vi "get_com_port.vi"(8 "error in (no error)":errorcluster, 11 "LightSourceAN191011Chameleon in":refnum<class "LightSourceAN191011Chameleon.lvclass">) -> (0 "error out":errorcluster, 2 "comm port":refnum<visa-resource-name>, 3 "LightSourceAN191011Chameleon out":refnum<class "LightSourceAN191011Chameleon.lvclass">)   [LabVIEW 2010, in "LightSourceAN191011Chameleon.lvclass"]
uses:
  LightSourceAN191011Chameleon.lvclass
  LightSourceAN191011Chameleon.lvclass/LightSourceAN191011Chameleon.ctl
  <vilib>/Instr/_visa.llb/VISA Configure Serial Port (Instr).vi
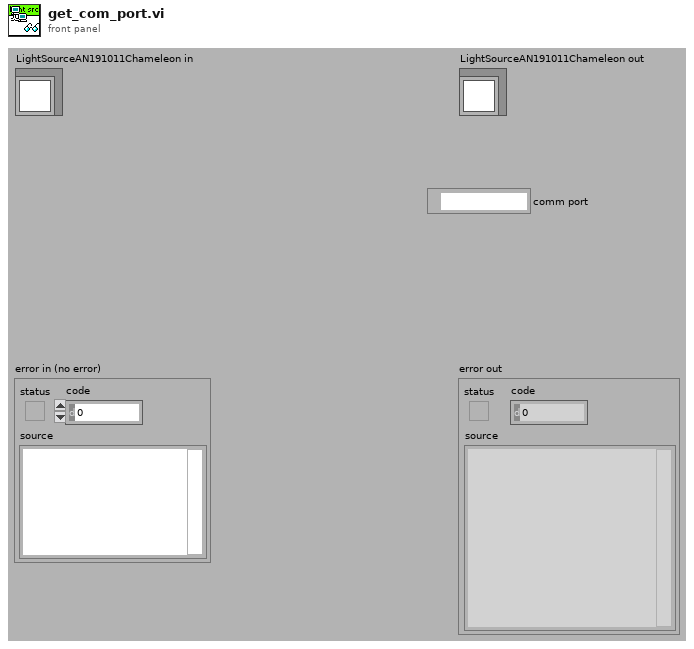
[diagram p1: front panel]
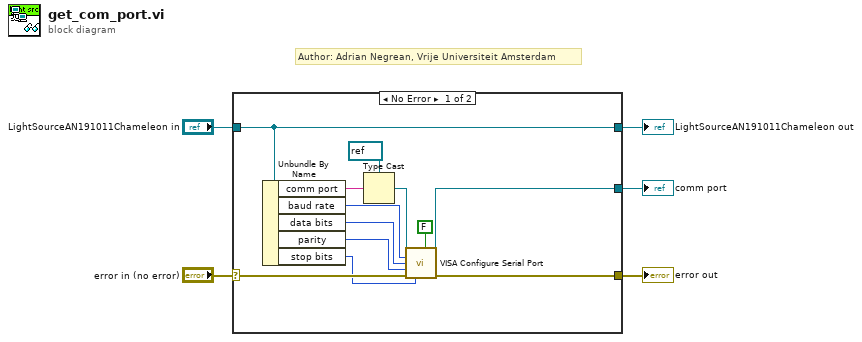
[diagram p0: block diagram]
diagram:
  # "Author: Adrian Negrean, Vrije Universiteit Amsterdam"
  n1 = case shown="No Error" "error in (no error)" {
    selector: "error in (no error)" -> [w7 w18]
    tunnel: [w13 w18] -> w4
    tunnel: [w17 w19] -> w2
    tunnel: "LightSourceAN191011Chameleon in" -> [w17 w19]
    tunnel: [w12 _] -> w1
    frame No Error {
      n2 = Unbundle By Name(w17) -> ("comm port"=w16:string, "baud rate"=w9:u32, "data bits"=w10:u16, "parity"=w11:enum16{"None", "Odd", "Even", "Mark", "Space"}, "stop bits"=w6:u16)
      n3 = Type Cast(type=refnum<visa-resource-name> refnum ("comm port"), x=w16) -> (*(type *) &x=w8:refnum<visa-resource-name>)
      n4 = call-poly "VISA Configure Serial Port"("VISA resource name"=w8, "Enable Termination\nChar (T)"=FALSE ("Enable Termination\nChar (T)"), "baud rate (9600)"=w9, "data bits (8)"=w10, "parity (0:none)"=w11, "error in (no error)"=w7, "stop bits (10: 1 bit)"=w6) -> ("VISA resource name out"=w12:refnum<visa-resource-name>, "error out"=w13:errorcluster)  [unwired: 7 in]
    }
    frame Error {
    }
  }
  "error out" <- w4
  "LightSourceAN191011Chameleon out" <- w2
  "comm port" <- w1
